vi "Дата_Время_проверка.vi"(9 "Целевое время":string, 10 "Целевая дата":string, 11 "Boolean 2":bool) -> (1 "Текущее время":string, 2 "Текущая дата":string, 3 "Boolean":bool)   [LabVIEW 2016]
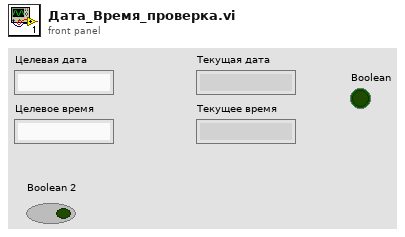
[diagram p1: front panel]
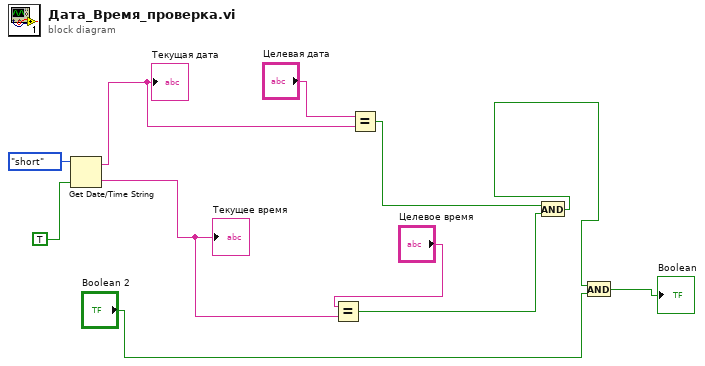
[diagram p0: block diagram]
diagram:
  n1 = Get Date/Time String(date format (0)=enum16{"short", "long", "abbreviated"}."short", want seconds? (F)=TRUE) -> (date string=w4:string, time string=w6:string)  [unwired: 1 in]
  "Текущая дата" <- w4
  "Текущее время" <- w6
  n2 = Equal?(x="Целевое время", y=w6) -> (x = y?=w7:bool)
  n3 = Equal?(x="Целевая дата", y=w4) -> (x = y?=w8:bool)
  n4 = And(x=w8, y=w7) -> (x .and. y?=w9:bool)
  n5 = And(x=w9, y="Boolean 2") -> (x .and. y?=→"Boolean":bool)
